vi "ResetInit.vi"(8 "error in":errorcluster) -> (0 "error out":errorcluster)   [LabVIEW 2014]
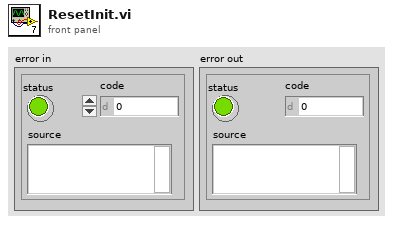
[diagram p1: front panel]
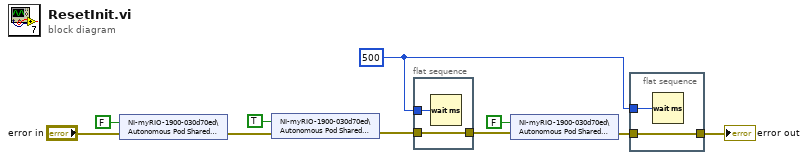
[diagram p0: block diagram]
diagram:
  w5 = u32 500 ("milliseconds to wait")
  n1 = shared-variable "NI-myRIO-1900-030d70ed\\Autonomous Pod Shared Variables.lvlib\\ResetSensor"(FALSE ("ResetSensor"), error in="error in") -> (error out=w7:errorcluster)
  n2 = shared-variable "NI-myRIO-1900-030d70ed\\Autonomous Pod Shared Variables.lvlib\\SensePower"(TRUE ("SensePower"), error in=w7) -> (error out=w4:errorcluster)
  n3 = flat-sequence {
    tunnel: w5 -> [w12]
    tunnel: w4 -> [w11]
    tunnel: [w11] -> w3
    frame #0 {
      n4 = Wait (ms)(milliseconds to wait=w12) -> ()  [unwired: 1 out]
    }
  }
  n5 = shared-variable "NI-myRIO-1900-030d70ed\\Autonomous Pod Shared Variables.lvlib\\SensePower"(FALSE ("SensePower"), error in=w3) -> (error out=w1:errorcluster)
  n6 = flat-sequence {
    tunnel: w5 -> [w14]
    tunnel: [w13] -> w2
    tunnel: w1 -> [w13]
    frame #0 {
      n7 = Wait (ms)(milliseconds to wait=w14) -> ()  [unwired: 1 out]
    }
  }
  "error out" <- w2
